vi "BRig_RT_loadData_startup.vi"(9 "input_dataMTrig":u16[](array[numeric]), 10 "input_dataLC":u16[](array[numeric]), 11 "input_dataExp":u16[](array[numeric])) -> (1 "output_dataMTrig":u16[](array[numeric]), 2 "output_dataLC":u16[](array[numeric]), 3 "output_dataExp":u16[](array[numeric]))   [LabVIEW 2014]
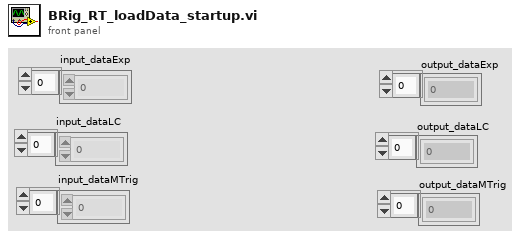
[diagram p1: front panel]
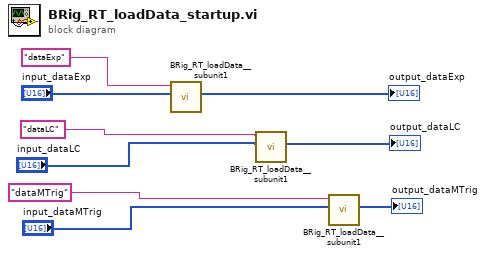
[diagram p0: block diagram]
diagram:
  n1 = call "BRig_RT_loadData__subunit1.vi"("input_data"="input_dataExp", "input_name"="dataExp" ("string")) -> ("output_data"=→"output_dataExp":u16[])  [unwired: 9 in]
  n2 = call "BRig_RT_loadData__subunit1.vi"("input_data"="input_dataLC", "input_name"="dataLC" ("string")) -> ("output_data"=→"output_dataLC":u16[])  [unwired: 9 in]
  n3 = call "BRig_RT_loadData__subunit1.vi"("input_data"="input_dataMTrig", "input_name"="dataMTrig" ("string")) -> ("output_data"=→"output_dataMTrig":u16[])  [unwired: 9 in]
